vi "draw.vi"(0 "reference":refnum<class "CallNode.lvclass">, 1 "graphics":refnum<class "Graphics.lvclass">, 5 "error in (no error)":errorcluster) -> (14 "reference out":refnum<class "CallNode.lvclass">, 19 "error out":errorcluster)   [LabVIEW 2020, in "CallNode.lvclass"]
uses:
  <resource>/Framework/Providers/Open_GDS/UML/CallNode_class/CallNode.lvclass
  C:/Program Files (x86)/National Instruments/LabVIEW 2020/resource/Framework/Providers/Open_GDS/UML/RectangularNode_class/RectangularNode.lvclass
  <resource>/Framework/Providers/Open_GDS/UML/Graphics_class/Graphics.lvclass
  <resource>/Framework/Providers/Open_GDS/UML/Graphics_class/StrokeType.ctl
  <resource>/Framework/Providers/Open_GDS/UML/General/Point/Point Point2D.ctl
  <resource>/Framework/Providers/Open_GDS/UML/RectangularNode_class/RectangularNode.lvclass
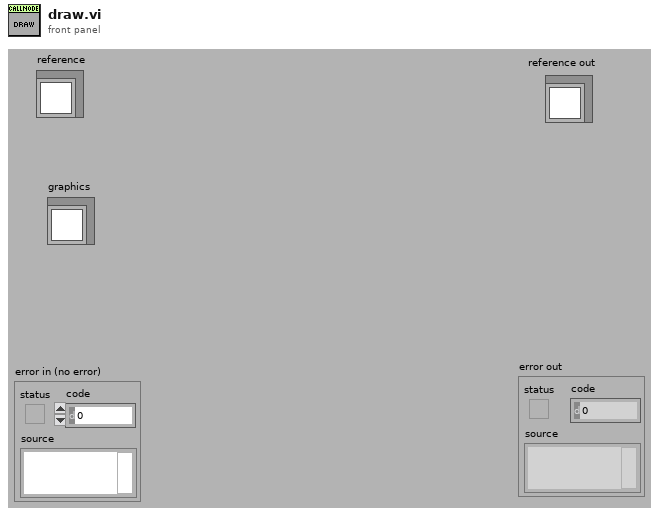
[diagram p1: front panel]
types:
  T1 = typedef "Graphics.lvclass/StrokeType.ctl" = enum16{"USE_DEFAULT", "SOLID", "DOTTED"}
  T2 = typedef "CallNode.lvclass/ObjectAttributes.ctl" = cluster{"objectCallNodeRef":refnum<class "AbstractNode.lvclass">, "signaled":bool, "openBottom":bool, "DEFAULT_WIDTH":i32, "DEFAULT_HEIGHT":i32, "CALL_YGAP":i32}
  T3 = typedef "RectangularNode.lvclass/ObjectAttributes.ctl" = cluster{"bounds":T4}
  T4 = typedef "Rectangle Rectangle2D.ctl" = cluster{"x":dbl, "y":dbl, "width":dbl, "height":dbl}
  T5 = typedef "Point Point2D.ctl" = cluster{"x":dbl, "y":dbl}
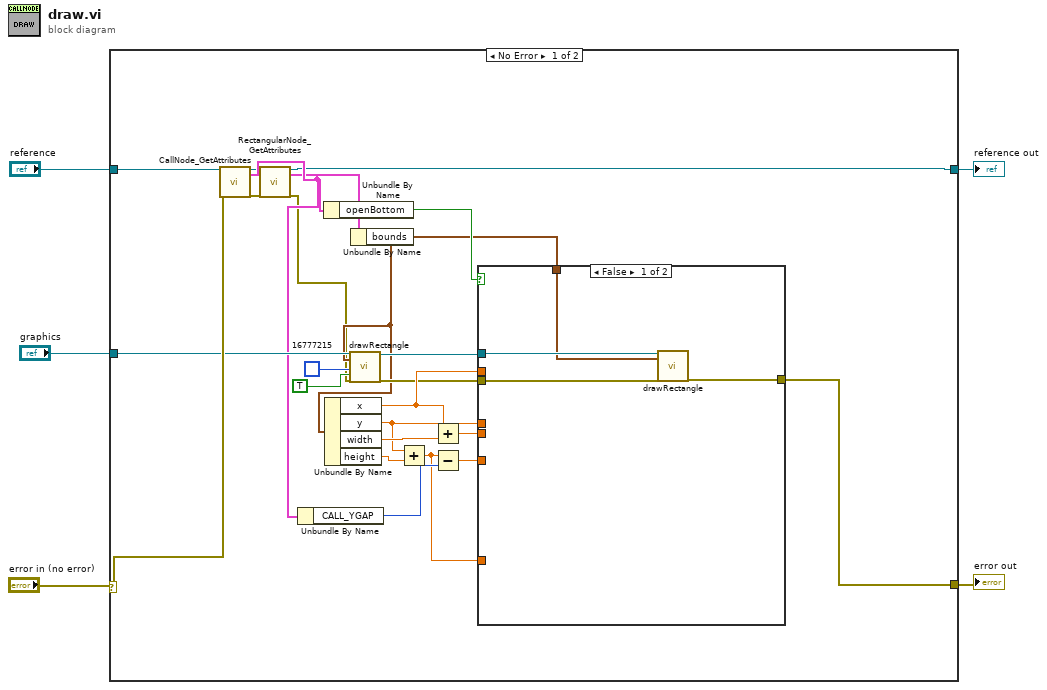
[diagram p0: block diagram]
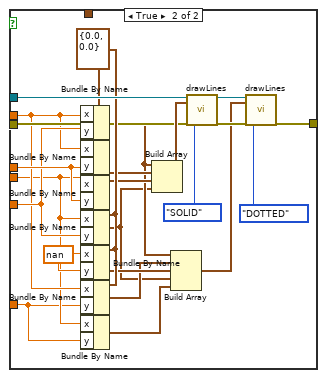
[diagram p2: hidden frame]
diagram:
  n1 = case shown="No Error" "error in (no error)" {
    selector: "error in (no error)" -> [w27 w57]
    tunnel: "reference" -> [w29 w58]
    tunnel: [w28 w57] -> w4
    tunnel: [w7 w58] -> w3
    tunnel: "graphics" -> [w26 _]
    frame No Error {
      n2 = call <resource>:"CallNode_GetAttributes.vi"("reference in"=w29, "error in (no error)"=w27) -> ("reference out"=w10:refnum<class "CallNode.lvclass">, "Data"=w11:T2, "error out"=w9:errorcluster)  [unwired: 1 in, 14 out]
      n3 = call <resource>:"RectangularNode_GetAttributes.vi"("reference in"=w10, "error in (no error)"=w9) -> ("reference out"=w7:refnum<class "CallNode.lvclass">, "Data"=w6:T3, "error out"=w8:errorcluster)  [unwired: 14 in, 1 out]
      n4 = Unbundle By Name(w11) -> ("CALL_YGAP"=w17:i32)
      n5 = Unbundle By Name(w11) -> ("openBottom"=w23:bool)
      n6 = Unbundle By Name(w6) -> ("bounds"=w12:T4)
      n7 = Unbundle By Name(w12) -> ("x"=w22:dbl, "y"=w19:dbl, "width"=w21:dbl, "height"=w18:dbl)
      n8 = call <resource>:"drawRectangle.vi"("reference"=w26, "rectangle"=w12, "color(if not used=default color)"=u32 16777215, "fill?(F)"=TRUE, "error in (no error)"=w8) -> ("reference out"=w13:refnum<class "Graphics.lvclass">, "error out"=w15:errorcluster)  [unwired: 2 in, 11 out]
      n9 = Add(x=w19, y=w18) -> (x+y=w14:dbl)
      n10 = Add(x=w22, y=w21) -> (x+y=w20:dbl)
      n11 = Subtract(x=w14, y=w17) -> (x-y=w16:dbl)
      n12 = case shown="False" w23 {
        tunnel: [w31 w56] -> w28
        tunnel: w13 -> [w32 w53]
        tunnel: w22 -> [_ w39]
        tunnel: w20 -> [_ w38]
        tunnel: w19 -> [_ w49]
        tunnel: w16 -> [_ w48]
        tunnel: w15 -> [w33 w44]
        tunnel: w14 -> [_ w34]
        tunnel: w12 -> [w30 _]
        frame False {
          n13 = call <resource>:"drawRectangle.vi"("reference"=w32, "rectangle"=w30, "error in (no error)"=w33) -> ("error out"=w31:errorcluster)  [unwired: 4 in, 12 out]
        }
        frame True {
          w50 = T5 {"x"=0.0, "y"=0.0} ("point2D")
          w40 = nan ("x")
          n14 = Bundle By Name(cluster=w50, "x"=w39, "y"=w48) -> (w42:T5)
          n15 = Bundle By Name(cluster=w50, "x"=w39, "y"=w49) -> (w47:T5)
          n16 = Bundle By Name(cluster=w50, "x"=w38, "y"=w49) -> (w46:T5)
          n17 = Bundle By Name(cluster=w50, "x"=w38, "y"=w48) -> (w36:T5)
          n18 = Bundle By Name(cluster=w50, "x"=w40, "y"=w40) -> (w41:T5)
          n19 = Bundle By Name(cluster=w50, "x"=w39, "y"=w34) -> (w37:T5)
          n20 = Bundle By Name(cluster=w50, "x"=w38, "y"=w34) -> (w35:T5)
          n21 = Build Array(w42, w47, w46, w36) -> (w45:T5[])
          n22 = Build Array(w42, w37, w41, w36, w35) -> (w43:T5[])
          n23 = call <resource>:"drawLines.vi"("reference"=w53, "points"=w45, "error in (no error)"=w44, "stroke"=StrokeType."SOLID") -> ("reference out"=w55:refnum<class "Graphics.lvclass">, "error out"=w54:errorcluster)  [unwired: 3 in, 11 out]
          n24 = call <resource>:"drawLines.vi"("reference"=w55, "points"=w43, "error in (no error)"=w54, "stroke"=StrokeType."DOTTED") -> ("error out"=w56:errorcluster)  [unwired: 3 in, 12 out]
        }
      }
    }
    frame Error {
    }
  }
  "reference out" <- w3
  "error out" <- w4
